vi "Temp Joystick.vi"(8 "error in (no error)":errorcluster, 9 "Fiducial?":bool, 10 "Component":T1, 11 "Gantry In":refnum<k24>) -> (0 "error out":errorcluster, 2 "Error?":bool, 3 "Gantry Out":refnum<k24>)   [LabVIEW 2021, in "Component Tray.lvclass"]
uses:
  Component Tray.lvclass
  Find Component.ctl
  Controller/Camera/Machine Vision.ctl
  C:/Program Files (x86)/Aerotech/A3200/LabVIEW/2010/Bin/Aerotech.A3200.dll
  Program Files (x86)/Aerotech/A3200/LabVIEW/2010/Bin/Aerotech.A3200.dll
  Component Tray.lvclass/Component Tray.ctl
  Controller/Motion/A3200/A3200.lvclass
  Controller/Camera/Camera.lvclass
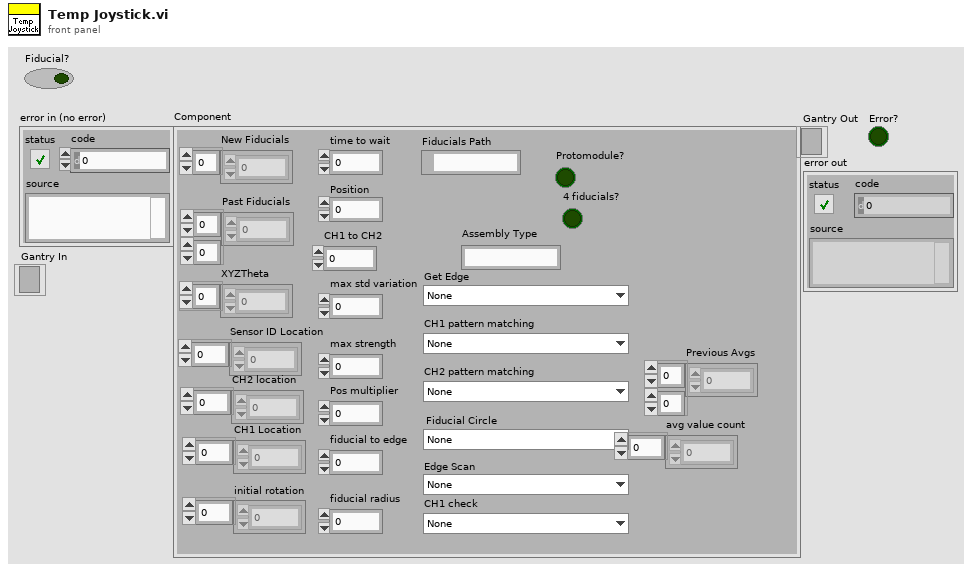
[diagram p1: front panel]
types:
  T1 = typedef "Component Tray.lvclass/Find Component.ctl" = cluster{"New Fiducials":dbl[], "Past Fiducials":dbl[][], "XYZTheta":dbl[], "Fiducials Path":path, "Position":i32, "CH1 Location":dbl[], "Sensor ID Location":dbl[], "initial rotation":dbl[], "CH2 location":dbl[], "max std variation":dbl, "max strength":dbl, "CH2 pattern matching":T2, "Fiducial Circle":T2, "Get Edge":T2, "Pos multiplier":dbl, "time to wait":u32, "fiducial to edge":dbl, "Protomodule?":bool, "Assembly Type":string, "CH1 to CH2":dbl, "Tray Number":string, "fiducial radius":dbl, "4 fiducials?":bool, "CH1 check":T2, "Edge Scan":T2, "CH1 pattern matching":T2, "Sensor Thickness":dbl, "Previous Avgs":dbl[][], "avg value count":dbl[]}
  T2 = typedef "Camera.lvclass/Machine Vision.ctl" = enum16{"None", "Assembly Tray Circle", "Assembly Tray Fiducial", "Partial Hexaboard", "sensor edge init", "HB edge init", "sensor edge pos1", "sensor edge pos2", "HB edge pos1", "HB edge pos2", "Sensor CH1-2", "HB CH1", "HB CH2", "V3 Sensor Circle", "Hexaboard Circle", "sensor CH1 check", "HB CH1 check ", "sensor ID"}
  T3 = typedef "File Paths.ctl" = cluster{"Glue Pattern Folder":path, "Carrier Tray Folder":path, "Pick Up Tool Fixture Folder":path, "Components Folder":path, "Bellows Tool Offset.txt":path, "Pick Up Tool Offset.txt":path, "Dispense Tip Offset.txt":path, "Log Files":path, "Gantry Assembly Map.txt":path, "Syringe and offset map.txt":path, "Controllers Folder":path, "Local dbase config":path}
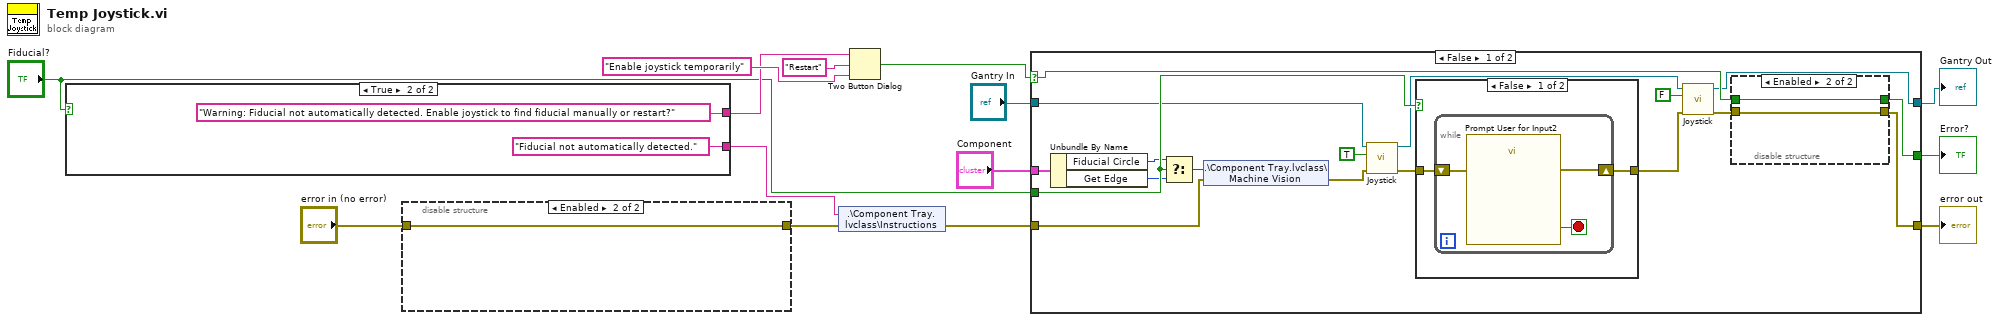
[diagram p0: block diagram]
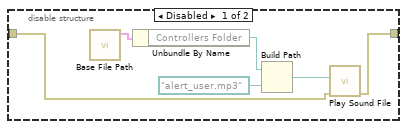
[diagram p2: hidden frame]
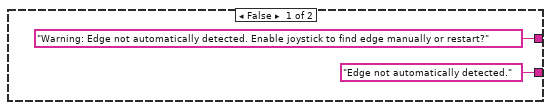
[diagram p3: hidden frame]
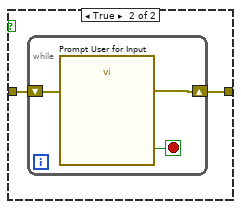
[diagram p4: hidden frame]
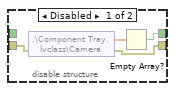
[diagram p5: hidden frame]
diagram:
  n1 = case shown="True" "Fiducial?" {
    tunnel: ["Warning: Edge not automatically detected. Enable joystick to find edge manually or restart?" ("message") "Warning: Fiducial not automatically detected. Enable joystick to find fiducial manually or restart?" ("message")] -> w5
    tunnel: ["Edge not automatically detected." ("Instructions") "Fiducial not automatically detected." ("Instructions")] -> w4
    frame False {
    }
    frame True {
    }
  }
  n2 = disable-structure shown="Enabled" {
    disable-tunnel: "error in (no error)" -> [w20 w25]
    disable-tunnel: [w19 w25] -> w1
    frame Disabled {
      n3 = call "Base File Path.vi"() -> ("Paths Out"=w22:T3)  [unwired: 11 in]
      n4 = Unbundle By Name(w22) -> ("Controllers Folder"=w24:path)
      n5 = Build Path(base path=w24, name or relative path=path "alert_user.mp3") -> (appended path=w23:path)
      n6 = call <vilib>:"Play Sound File.vi"("error in (no error)"=w20, "path"=w23) -> ("error out"=w19:errorcluster)  [unwired: 8 in, 1 out]
    }
    frame Enabled {
    }
  }
  n7 = shared-variable ".\\Component Tray.lvclass\\Instructions"(w4, error in=w1) -> (error out=w14:errorcluster)
  n8 = Two Button Dialog(message=w5, 1:"Enable joystick temporarily" ("F button name (\"Cancel\")"), 2:"Restart" ("T button name (\"OK\")")) -> (T button?=w6:bool)
  n9 = case shown="False" w6 {
    selector: w6 -> [w38 w60]
    tunnel: "Gantry In" -> [w37 w62]
    tunnel: [w35 w62] -> w11
    tunnel: w14 -> [w42 w61]
    tunnel: [w41 w61] -> w10
    tunnel: "Component" -> [w43 _]
    tunnel: [w40 w60] -> w9
    tunnel: "Fiducial?" -> [w39 _]
    frame False {
      n10 = Unbundle By Name(w43) -> ("Fiducial Circle"=w28:T2, "Get Edge"=w26:T2)
      n11 = Select(t=w28, s=w39, f=w26) -> (s? t:f=w27:T2)
      n12 = shared-variable ".\\Component Tray.lvclass\\Machine Vision"(w27, error in=w42) -> (error out=w34:errorcluster)
      n13 = call "Joystick.vi"("error in (no error)"=w34, "Joystick"=TRUE, "Gantry In"=w37) -> ("error out"=w32:errorcluster, "Gantry Out"=w29:refnum<k24>)  [unwired: 7 in]
      n14 = case shown="False" w39 {
        tunnel: w32 -> [w44 w50]
        tunnel: [w45 w49] -> w31
        frame False {
          n15 = while {
            shift-right: [w47] -> w45
            shift-left: w44 -> [w48]
            stop <- w46 stop-if-true
            n16 = call "Prompt User for Input2"("error in (no error)"=w48) -> ("Target lined up?"=w46:bool, "error out"=w47:errorcluster)  [unwired: 16 in, 1 out]
          }
        }
        frame True {
          n17 = while {
            shift-right: [w52] -> w49
            shift-left: w50 -> [w53]
            stop <- w51 stop-if-true
            n18 = call "Prompt User for Input"("error in (no error)"=w53) -> ("Target lined up?"=w51:bool, "error out"=w52:errorcluster)  [unwired: 16 in, 1 out]
          }
        }
      }
      n19 = call "Joystick.vi"("error in (no error)"=w31, "Joystick"=FALSE, "Gantry In"=w29) -> ("error out"=w36:errorcluster, "Gantry Out"=w35:refnum<k24>)  [unwired: 7 in]
      n20 = disable-structure shown="Enabled" {
        disable-tunnel: w36 -> [w56 w59]
        disable-tunnel: [w55 w59] -> w41
        disable-tunnel: [w54 w58] -> w40
        disable-tunnel: w38 -> [_ w58]
        frame Disabled {
          n21 = shared-variable ".\\Component Tray.lvclass\\Camera"(error in=w56) -> (w57:dbl[], error out=w55:errorcluster)
          n22 = Empty Array?(array=w57) -> (empty?=w54:bool)
        }
        frame Enabled {
        }
      }
    }
    frame True {
    }
  }
  "Gantry Out" <- w11
  "error out" <- w10
  "Error?" <- w9
